vi "Start Stop Laser Example.vi"() -> ()   [LabVIEW 2019]
uses:
  C:/Users/tim/Documents/kSAComm LabView Sample/kSACommInterface.dll
  kSACommInterface.dll
  <vilib>/regexp/Match Regular Expression.xnode
panel:
  out "Connected":bool
  in  "IP Address":string="192.168.0.169"
  in  "Exit":bool
  in  "Laser On/Off":bool
  # "Upon starting this VI a connection will be made to a kSA application running on a PC using this IP address. The LED indicates successful connection."
  # "Press this button to turn the laser \"On\"  or \"Off\" in the kSA application. The LED inside the button will indicate whether or not the laser is currently \"On\" or \"Off\"."
  # "Press this button to cleanly disconnect from the kSA application and exit the VI"
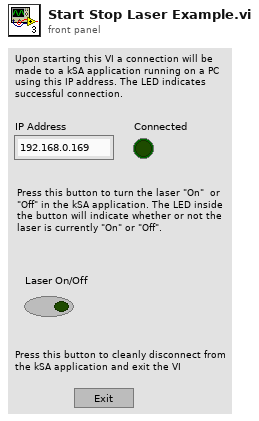
[diagram p1: front panel]
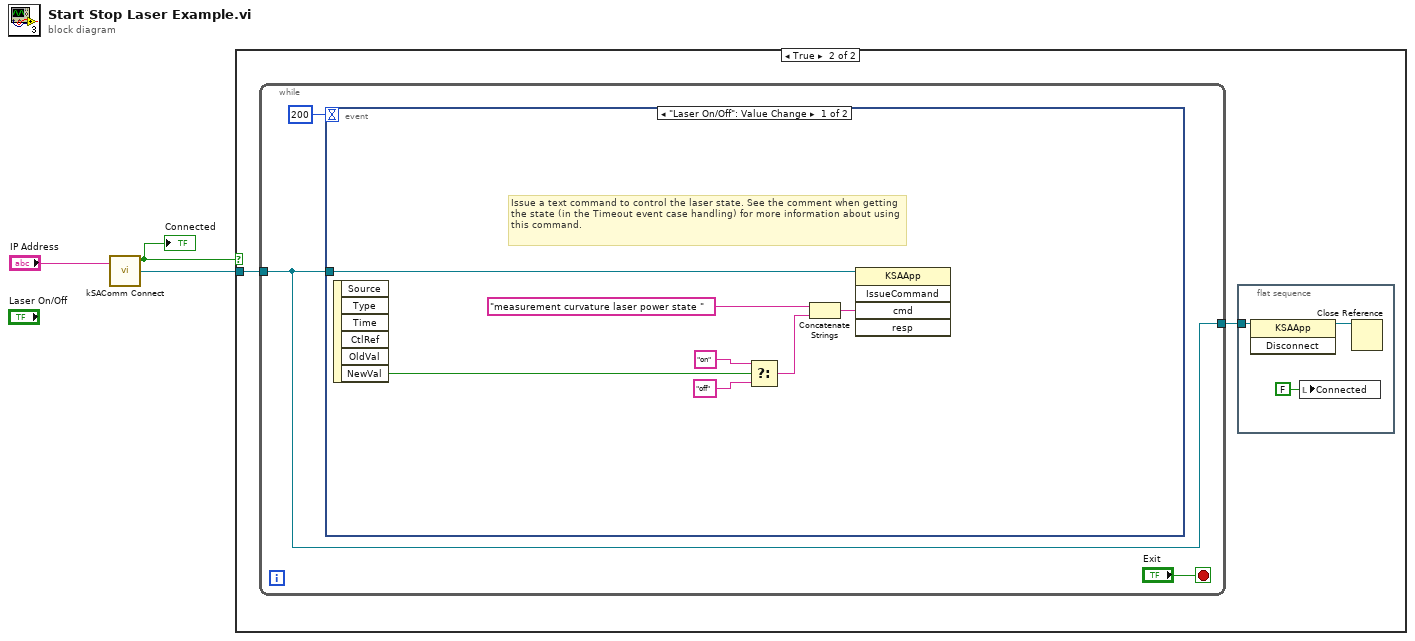
[diagram p0: block diagram]
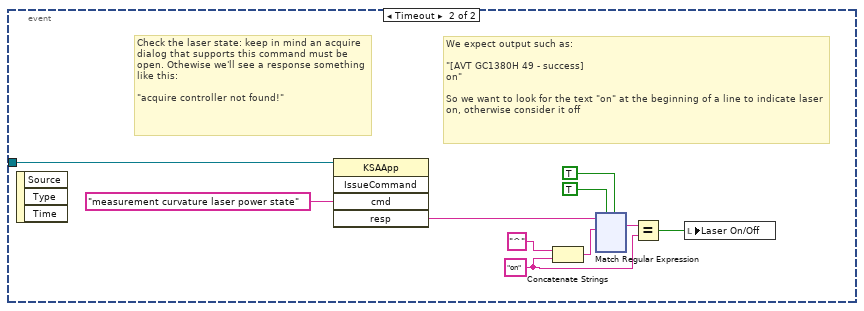
[diagram p3: hidden frame]
diagram:
  n1 = call "kSAComm Connect.vi"("IP Address"="IP Address") -> ("Connect"=w1:bool, "kSAComm ref out"=w2:refnum<k24>)  [unwired: 2 in]
  "Connected" <- w1
  n2 = case shown="True" w1 {
    tunnel: w2 -> [_ w5]
    frame False {
    }
    frame True {
      n3 = while {
        tunnel: w5 -> [w9]
        tunnel: [w9] -> w4
        stop <- "Exit" stop-if-true
        n4 = event shown="[0] \"Laser On/Off\": Value Change" {
          selector: _ -> [_ _]
          dyn-events: _ -> [_ _]
          timeout: 200 -> [_ _]
          tunnel: w9 -> [w13 w20]
          event "Laser On/Off": Value Change {
            # "Issue a text command to control the laser state. See the comment when getting the state (in the Timeout event case handling) for more information about using this command."
            n5 = event-data() -> ("NewVal"=w12:bool)  [unwired: 1 in, 5 out]
            n6 = Select(t="on", s=w12, f="off") -> (s? t:f=w15:string)
            n7 = Concatenate Strings("measurement curvature laser power state ", w15) -> (w14:string)
            n8 = invoke class="KSAApp" method="IssueCommand"(reference=w13, "cmd"=w14) -> ()  [unwired: 3 in, 5 out]
          }
          event Timeout {
            w24 = "on" ("regular expression")
            # "Check the laser state: keep in mind an acquire dialog that supports this command must be open. Othewise we'll see a response something like this:\n\n\"acquire controller not found!\""
            # "We expect output such as:\n\n\"[AVT GC1380H 49 - success]\non\"\n\nSo we want to look for the text \"on\" at the beginning of a line to indicate laser on, otherwise consider it off"
            n9 = event-data() -> ()  [unwired: 1 in, 3 out]
            n10 = invoke class="KSAApp" method="IssueCommand"(reference=w20, "cmd"="measurement curvature laser power state") -> ("resp"=w26:string)  [unwired: 3 in, 4 out]
            n11 = Concatenate Strings("^", w24) -> (w28:string)
            n12 = xnode "Match Regular Expression"("input string"=w26, "regular expression"=w28, "ignore case? (F)"=TRUE, "multiline? (F)"=TRUE) -> ("whole match"=w27:string)  [unwired: 2 in, 4 out]
            n13 = Equal?(x=w27, y=w24) -> (x = y?=w19:bool)
            n14 = local write "Laser On/Off"(w19) -> ()
          }
        }
      }
      n15 = flat-sequence {
        tunnel: w4 -> [w7]
        frame #0 {
          n16 = invoke class="KSAApp" method="Disconnect"(reference=w7) -> (reference out=w8:refnum<k24>)  [unwired: 2 in, 2 out]
          n17 = local write "Connected"(FALSE ("Connected")) -> ()
          n18 = Close Reference(reference=w8) -> ()  [unwired: 1 in, 1 out]
        }
      }
    }
  }
